vi "T7 Process Stream Data KAG.vi"(7 "Backlog":bool, 8 "error in":errorcluster, 9 "TCP Data In":string, 10 "Stream Configuration":T3={"Scan Rate (Hz)"=1000.0, "Samples Per Packet"=512, "Resolution Index"=0, "Buffer Size (bytes)"=32768, "NumScans"=1500, "Read Timeout (ms)"=5000.0, "Scan Table"=[{"Channel"=0, "BipGain"=0, "Input Config"="Single-Ended"}, {"Channel"=1, "BipGain"=0, "Input Config"="Single-Ended"}, {"Channel"=2, "BipGain"=0, "Input Config"="Single-Ended"}, {"Channel"=3, "BipGain"=0, "Input Config"="Single-Ended"}]} {"Samples Per Packet" max=512 step=1; "Buffer Size (bytes)" max=32768 step=1; "Resolution Index" max=8 step=1; "Scan Rate (Hz)" min=0.0 max=100000.0; "Scan Table"."BipGain" items=["x1", "x10", "x100", "x1000"]; "Scan Table"."Channel" step=1}, 11 "IP Configuration":T1={"Connection ID In"=refnum, "Connection ID Out"=refnum, "Device IP"="192.168.126.147", "Port"=502}) -> (0 "error out":errorcluster, 1 "Backlog Bytes":u16, 3 "Data":u16[][](array[numeric]), 5 "Packet Counter Out":i32)   [LabVIEW 2015]
doc: "Check Packet integrity and parse"
uses:
  T7 Stream Config KAG.ctl
  T7 Secondary Configs KAG.ctl
  T7 IP Config KAG.ctl
  T7 Stream Globals KAG.vi
panel:
  in  "Secondary Stream Configurations":T2={"Settling Delay (*5 us)"=0.0, "Clock Source"=0, "Auto Target"=1} {"Auto Target" max=255 step=1; "Clock Source" max=2 step=2; "Settling Delay (*5 us)" min=0.0 max=5000.0 step=1.0}
  in  "Tab Control":T4(tab)=enum."Data Array"
  out "Read Array":u8[](array[numeric]) format="%.0x"
  out "# of bytes received":i32
  out "# Bytes to Read":i32
  out "Sample Interval":dbl
  in  "Samples per Channel":i32
  out "Backlog Scans":dbl
  out "# packets":i32
  out "scans/packet":i32[](array[numeric])
  out "unsigned byte array":u8[](array[numeric])
  out "ErrorBoolean":bool
  out "Bytes / Pkt":u32
  out "Error Array":i32[][](array[numeric])
  # "29 October 2015 --\n\nI changed the VI execution from \"preallocated clone reentrant execution\" to \"Non-reentrant execution\"  while I am debugging. May want to change that back before deployment."
  # "Transaction ID"
  # "Protocol ID"
  # "Length"
  # "1 (Unit ID)"
  # "76 (Function)"
  # "Number of Samples in Current Read"
  # "Backlog"
  # "Status Code"
  # "Additional Status Info"
  # "Stream Data"
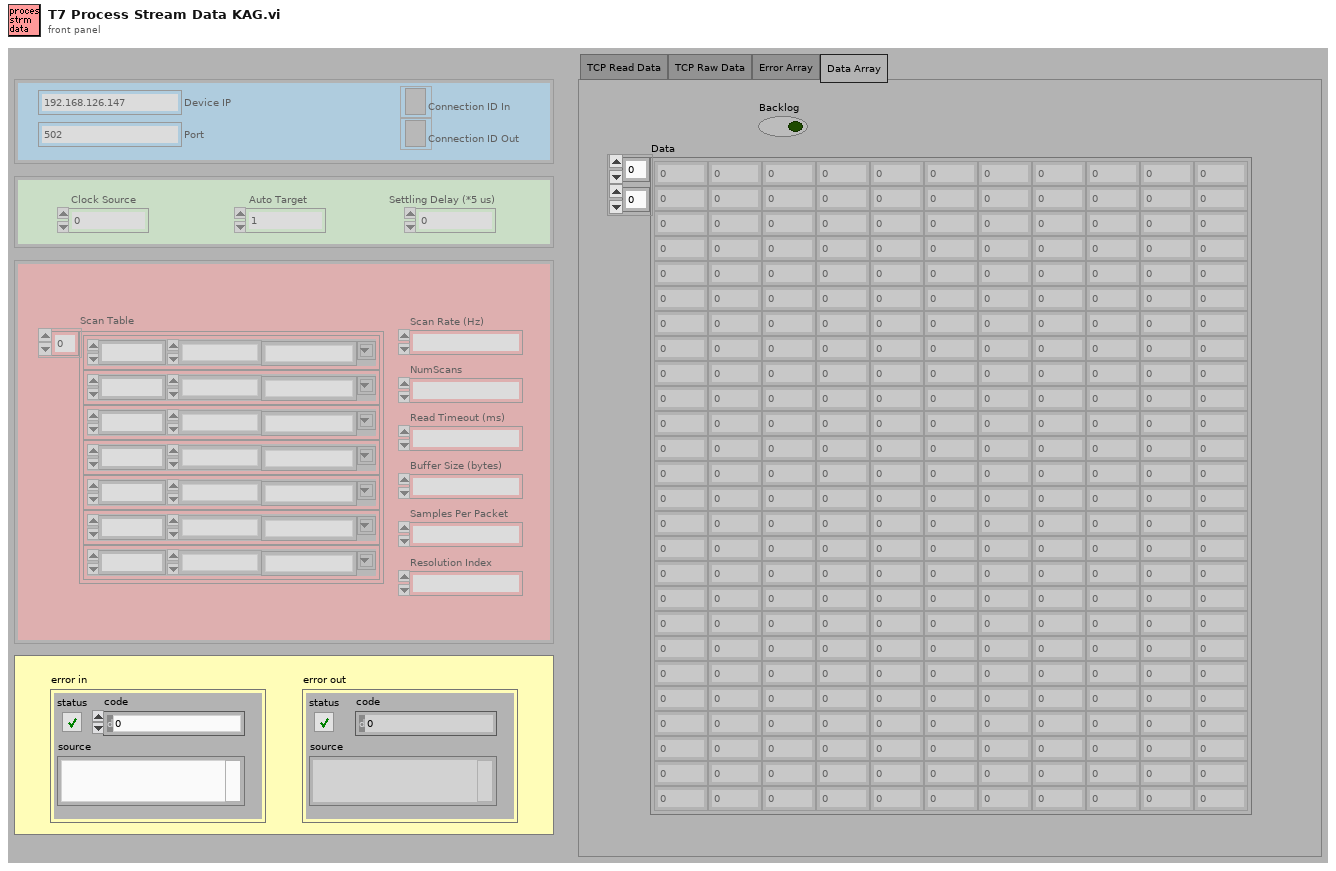
[diagram p1: front panel]
types:
  T1 = typedef "T7 IP Config KAG.ctl" = cluster{"Connection ID In":refnum<k5>, "Connection ID Out":refnum<k5>, "Device IP":string, "Port":i32}
  T2 = typedef "T7 Secondary Configs KAG.ctl" = cluster{"Settling Delay (*5 us)":dbl, "Clock Source":u32, "Auto Target":u32}
  T3 = typedef "T7 Stream Config KAG.ctl" = cluster{"Scan Rate (Hz)":dbl, "Samples Per Packet":u32, "Resolution Index":u32, "Buffer Size (bytes)":u32, "NumScans":u32, "Read Timeout (ms)":dbl, "Scan Table":cluster{"Channel":u32, "BipGain":u32, "Input Config":string}[]}
  T4 = enum32{"TCP Read Data", "TCP Raw Data", "Error Array", "Data Array"}
  T5 = cluster{"Channel":u32, "BipGain":u32, "Input Config":string}[]
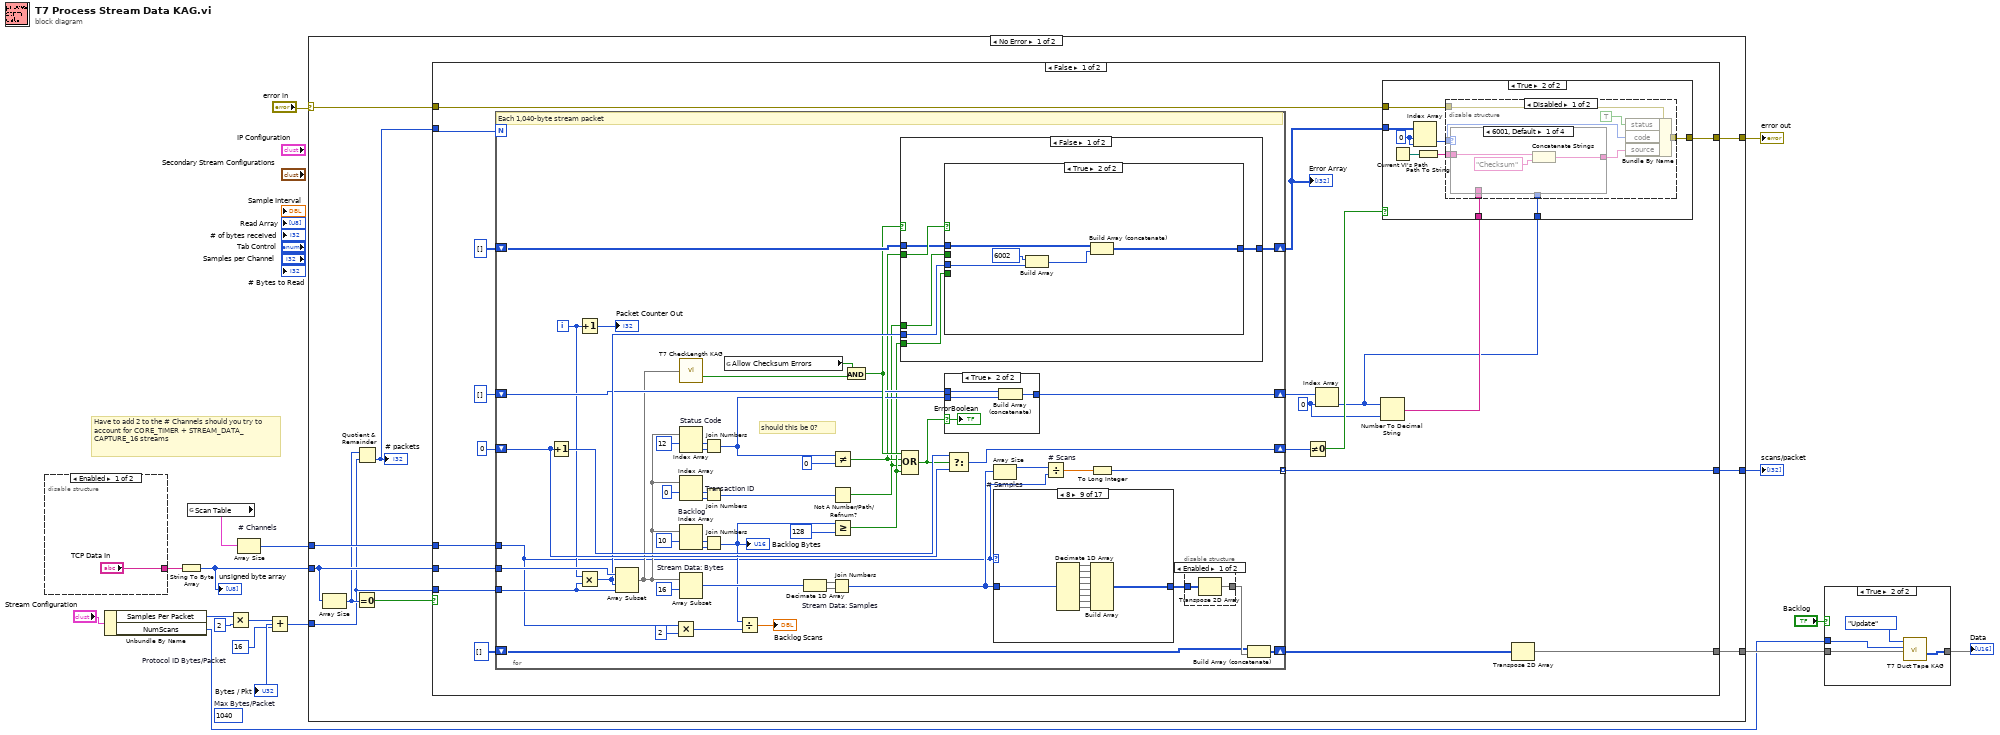
[diagram p0: block diagram]
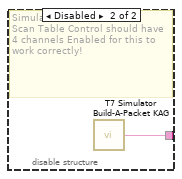
[diagram p3: hidden frame]
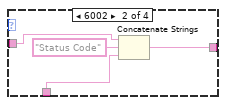
[diagram p5: hidden frame]
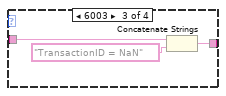
[diagram p6: hidden frame]
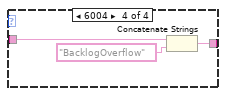
[diagram p7: hidden frame]
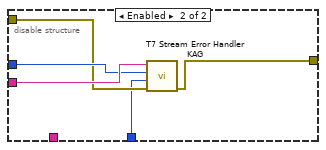
[diagram p8: hidden frame]
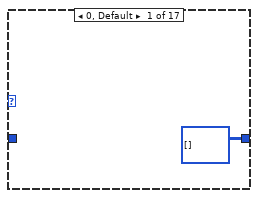
[diagram p10: hidden frame]
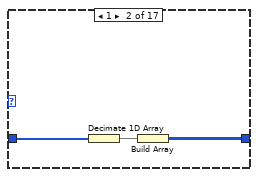
[diagram p11: hidden frame]
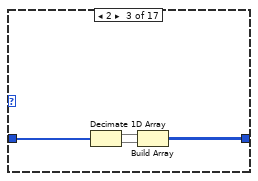
[diagram p12: hidden frame]
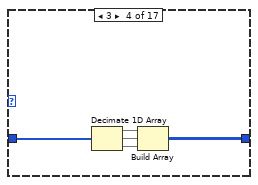
[diagram p13: hidden frame]
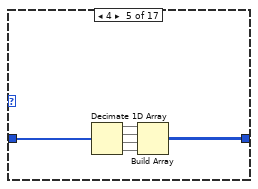
[diagram p14: hidden frame]
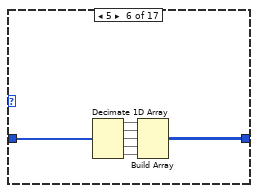
[diagram p15: hidden frame]
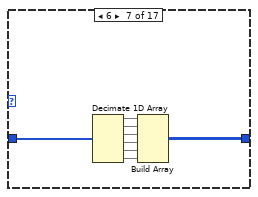
[diagram p16: hidden frame]
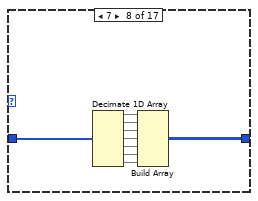
[diagram p17: hidden frame]
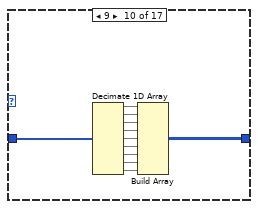
[diagram p18: hidden frame]
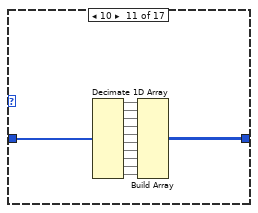
[diagram p19: hidden frame]
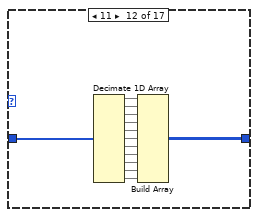
[diagram p20: hidden frame]
diagram:
  w5 = 16  # Protocol ID Bytes/Packet
  (unwired) 1040  # Max Bytes/Packet
  # "Have to add 2 to the # Channels should you try to account for CORE_TIMER + STREAM_DATA_CAPTURE_16 streams"
  n1 = disable-structure shown="Enabled" {
    disable-tunnel: ["TCP Data In" w19] -> w17
    frame Enabled {
    }
    frame Disabled {
      # "Simulate Packet\nScan Table Control should have 4 channels Enabled for this to work correctly!"
      n2 = call "T7 Simulator Build-A-Packet KAG.vi"() -> ("Simulated Data Packet"=w19:string)  [unwired: 10 in]
    }
  }
  n3 = Unbundle By Name("Stream Configuration") -> ("Samples Per Packet"=w8:u32, "NumScans"=w2:u32)
  n4 = String To Byte Array(string=w17) -> (unsigned byte array=w16:u8[])
  "unsigned byte array" <- w16
  n5 = global read "T7 Stream Globals KAG.vi" "Scan Table"() -> (w12:T5)
  n6 = Multiply(x=w8, y=2) -> (x*y=w6:u32)
  n7 = Array Size "# Channels"(array=w12) -> (size(s)=w11:i32)
  n8 = Add(x=w6, y=w5) -> (x+y=w7:u32)
  "Bytes / Pkt" <- w7
  n9 = case shown="No Error" "error in" {
    selector: "error in" -> [w29 w358]
    tunnel: [w28 w358] -> w13
    tunnel: w16 -> [w27 _]
    tunnel: w11 -> [w26 _]
    tunnel: [w25 u16[][] []] -> w4
    tunnel: w7 -> [w23 _]
    tunnel: [w21 i32[] []] -> w15
    frame No Error {
      n10 = Array Size(array=w27) -> (size(s)=w24:i32)
      n11 = Equal To 0?(x=w24) -> (x = 0?=w22:bool)
      n12 = Quotient & Remainder(x=w24, y=w23) -> (floor(x/y)=w20:u32)  [unwired: 1 out]
      "# packets" <- w20
      n13 = case shown="False" w22 {
        tunnel: w27 -> [w49 _]
        tunnel: w20 -> [w39 _]
        tunnel: w23 -> [w48 _]
        tunnel: w29 -> [w46 w352]
        tunnel: [w43 w351] -> w28
        tunnel: w26 -> [w40 _]
        tunnel: [w30 u16[][] []] -> w25
        tunnel: [w35 i32[] []] -> w21
        frame False {
          w34 = 0 ("Index")
          n14 = for {
            N: w39 -> [_]
            tunnel: w49 -> [w134]
            tunnel: w48 -> [w94]
            shift-right: [w132] -> w45
            shift-left: 0 -> [w133]
            shift-right: [w130] -> w41
            shift-left: i32[][] [] -> [w131]
            tunnel: w40 -> [w90]
            shift-right: [w119] -> w37
            shift-left: u16[] [] -> [w120]
            tunnel: [w100] -> w35 mode=indexing
            shift-right: [w86] -> w31
            shift-left: u16[][] [] -> [w85]
            i -> [w95]
            # "should this be 0?"
            # "Each 1,040-byte stream packet"
            n15 = Increment(x=w133) -> (x+1=w129:i32)
            n16 = Increment(x=w95) -> (x+1=→"Packet Counter Out":i32)
            n17 = Multiply(x=w95, y=w94) -> (x*y=w124:u32)
            n18 = Array Subset(array=w134, index=w124, length=w94) -> (w116:u8[])
            n19 = Multiply(x=w90, y=2) -> (x*y=w91:i32)
            n20 = call "T7 CheckLength KAG.vi"("Array"=w116) -> ("CheckLength Error"=w117:bool)  [unwired: 1 out]
            n21 = Index Array "Status Code"(array=w116, index #1=12 ("Index")) -> (element #1=w115:u8, element #2=w114:u8)  [unwired: 1 in]
            n22 = Index Array "Transaction ID"(array=w116, index #1=0 ("Index")) -> (element #1=w111:u8, element #2=w112:u8)  [unwired: 1 in]
            n23 = Index Array "Backlog"(array=w116, index #1=10 ("Index")) -> (element #1=w108:u8, element #2=w109:u8)  [unwired: 1 in]
            n24 = Array Subset "Stream Data: Bytes"(array=w116, index=16 ("Array Index")) -> (w107:u8[])  [unwired: 1 in]
            n25 = Join Numbers(hi=w115, lo=w114) -> ((hi.lo)=w113:u16)
            n26 = Join Numbers(hi=w111, lo=w112) -> ((hi.lo)=w110:u16)
            n27 = Join Numbers(hi=w108, lo=w109) -> ((hi.lo)=w92:u16)
            "Backlog Bytes" <- w92
            n28 = global read "T7 Stream Globals KAG.vi" "Allow Checksum Errors"() -> (w93:bool)
            n29 = Divide(x=w92, y=w91) -> (x/y=→"Backlog Scans":dbl)
            n30 = Decimate 1D Array(w107) -> (w106:u8[], w105:u8[])
            n31 = Join Numbers "Stream Data: Samples"(hi=w106, lo=w105) -> ((hi.lo)=w104:u16[])
            n32 = Not Equal?(x=w113, y=u16 0) -> (x != y?=w97:bool)
            n33 = Not A Number/Path/Refnum?(number/path/refnum=w110) -> (NaN/Path/Refnum?=w96:bool)
            n34 = Greater Or Equal?(x=w92, y=u8 128) -> (x >= y?=w98:bool)
            n35 = And(x=w93, y=w117) -> (x .and. y?=w121:bool)
            n36 = case shown="False" w121 {
              tunnel: w97 -> [w317 _]
              tunnel: w96 -> [w316 _]
              tunnel: w124 -> [w315 w346]
              tunnel: w131 -> [w313 w345]
              tunnel: [w314 w343] -> w130
              tunnel: w98 -> [w312 _]
              frame False {
                n37 = case shown="True" w317 {
                  tunnel: w316 -> [w322 _]
                  tunnel: w315 -> [w321 w340]
                  tunnel: [w319 w339] -> w314
                  tunnel: w313 -> [w320 w338]
                  tunnel: w312 -> [w318 _]
                  frame False {
                    n38 = case shown="True" w322 {
                      tunnel: w321 -> [w325 w335]
                      tunnel: w320 -> [w326 w334]
                      tunnel: [w324 w333] -> w319
                      tunnel: w318 -> [w323 _]
                      frame False {
                        n39 = case shown="True" w323 {
                          tunnel: w326 -> [w327 w330]
                          tunnel: [w327 w328] -> w324
                          tunnel: w325 -> [_ w329]
                          frame False {
                          }
                          frame True {
                            n40 = Build Array(6004, w329) -> (w331:u32[])
                            n41 = Build Array (concatenate)(w330, w331) -> (w328:u32[][])
                          }
                        }
                      }
                      frame True {
                        n42 = Build Array(6003, w335) -> (w336:u32[])
                        n43 = Build Array (concatenate)(w334, w336) -> (w333:u32[][])
                      }
                    }
                  }
                  frame True {
                    n44 = Build Array(6002, w340) -> (w341:u32[])
                    n45 = Build Array (concatenate)(w338, w341) -> (w339:u32[][])
                  }
                }
              }
              frame True {
                n46 = Build Array(6001, w346) -> (w344:u32[])
                n47 = Build Array (concatenate)(w345, w344) -> (w343:u32[][])
              }
            }
            n48 = Compound Arithmetic op=OR(w121, w97, w96, w98) -> (w122:bool)
            n49 = case shown="True" w122 {
              selector: w122 -> [_ w311]
              tunnel: w113 -> [_ w310]
              tunnel: w120 -> [w307 w309]
              tunnel: [w307 w308] -> w119
              frame False {
              }
              frame True {
                n50 = Build Array (concatenate)(w309, w310) -> (w308:u16[])
                "ErrorBoolean" <- w311
              }
            }
            n51 = Select(t=w129, s=w122, f=w133) -> (s? t:f=w132:i32)
            n52 = Array Size "# Samples"(array=w104) -> (size(s)=w102:i32)
            n53 = case shown="8" w90 {
              tunnel: w104 -> [_ w141 w145 w150 w156 w163 w171 w180 w190 w201 w213 w226 w240 w255 w271 w288 w306]
              tunnel: [u16[][] [] w139 w142 w146 w151 w157 w164 w172 w181 w191 w202 w214 w227 w242 w258 w275 w293] -> w103
              frame 0, Default {
              }
              frame 1 {
                n54 = Decimate 1D Array(w141) -> (w140:u16[])
                n55 = Build Array(w140) -> (w139:u16[][])
              }
              frame 2 {
                n56 = Decimate 1D Array(w145) -> (w144:u16[], w143:u16[])
                n57 = Build Array(w144, w143) -> (w142:u16[][])
              }
              frame 3 {
                n58 = Decimate 1D Array(w150) -> (w149:u16[], w148:u16[], w147:u16[])
                n59 = Build Array(w149, w148, w147) -> (w146:u16[][])
              }
              frame 4 {
                n60 = Decimate 1D Array(w156) -> (w155:u16[], w154:u16[], w153:u16[], w152:u16[])
                n61 = Build Array(w155, w154, w153, w152) -> (w151:u16[][])
              }
              frame 5 {
                n62 = Decimate 1D Array(w163) -> (w162:u16[], w161:u16[], w160:u16[], w159:u16[], w158:u16[])
                n63 = Build Array(w162, w161, w160, w159, w158) -> (w157:u16[][])
              }
              frame 6 {
                n64 = Decimate 1D Array(w171) -> (w170:u16[], w169:u16[], w168:u16[], w167:u16[], w166:u16[], w165:u16[])
                n65 = Build Array(w170, w169, w168, w167, w166, w165) -> (w164:u16[][])
              }
              frame 7 {
                n66 = Decimate 1D Array(w180) -> (w179:u16[], w178:u16[], w177:u16[], w176:u16[], w175:u16[], w174:u16[], w173:u16[])
                n67 = Build Array(w179, w178, w177, w176, w175, w174, w173) -> (w172:u16[][])
              }
              frame 8 {
                n68 = Decimate 1D Array(w190) -> (w189:u16[], w188:u16[], w187:u16[], w186:u16[], w185:u16[], w184:u16[], w183:u16[], w182:u16[])
                n69 = Build Array(w189, w188, w187, w186, w185, w184, w183, w182) -> (w181:u16[][])
              }
              frame 9 {
                n70 = Decimate 1D Array(w201) -> (w200:u16[], w199:u16[], w198:u16[], w197:u16[], w196:u16[], w195:u16[], w194:u16[], w193:u16[], w192:u16[])
                n71 = Build Array(w200, w199, w198, w197, w196, w195, w194, w193, w192) -> (w191:u16[][])
              }
              frame 10 {
                n72 = Decimate 1D Array(w213) -> (w212:u16[], w211:u16[], w210:u16[], w209:u16[], w208:u16[], w207:u16[], w206:u16[], w205:u16[], w204:u16[], w203:u16[])
                n73 = Build Array(w212, w211, w210, w209, w208, w207, w206, w205, w204, w203) -> (w202:u16[][])
              }
              frame 11 {
                n74 = Decimate 1D Array(w226) -> (w225:u16[], w224:u16[], w223:u16[], w222:u16[], w221:u16[], w220:u16[], w219:u16[], w218:u16[], w217:u16[], w216:u16[], w215:u16[])
                n75 = Build Array(w225, w224, w223, w222, w221, w220, w219, w218, w217, w216, w215) -> (w214:u16[][])
              }
              frame 12 {
                n76 = Decimate 1D Array(w240) -> (w239:u16[], w238:u16[], w237:u16[], w236:u16[], w235:u16[], w234:u16[], w233:u16[], w232:u16[], w231:u16[], w230:u16[], w229:u16[], w228:u16[])
                n77 = Build Array(w239, w238, w237, w236, w235, w234, w233, w232, w231, w230, w229, w228) -> (w227:u16[][])
              }
              frame 13 {
                n78 = Decimate 1D Array(w255) -> (w254:u16[], w253:u16[], w252:u16[], w251:u16[], w250:u16[], w249:u16[], w248:u16[], w247:u16[], w246:u16[], w245:u16[], w244:u16[], w243:u16[], w241:u16[])
                n79 = Build Array(w254, w253, w252, w251, w250, w249, w248, w247, w246, w245, w244, w243, w241) -> (w242:u16[][])
              }
              frame 14 {
                # "Unless AI is expanded with MUX 80, max AIN = 14"
                n80 = Decimate 1D Array(w271) -> (w270:u16[], w269:u16[], w268:u16[], w267:u16[], w266:u16[], w265:u16[], w264:u16[], w263:u16[], w262:u16[], w261:u16[], w260:u16[], w259:u16[], w257:u16[], w256:u16[])
                n81 = Build Array(w270, w269, w268, w267, w266, w265, w264, w263, w262, w261, w260, w259, w257, w256) -> (w258:u16[][])
              }
              frame 15 {
                # "Added this to account for CORE_TIMER stream"
                n82 = Decimate 1D Array(w288) -> (w287:u16[], w286:u16[], w285:u16[], w284:u16[], w283:u16[], w282:u16[], w281:u16[], w280:u16[], w279:u16[], w278:u16[], w277:u16[], w276:u16[], w274:u16[], w273:u16[], w272:u16[])
                n83 = Build Array(w287, w286, w285, w284, w283, w282, w281, w280, w279, w278, w277, w276, w274, w273, w272) -> (w275:u16[][])
              }
              frame 16 {
                # "Added this to account for STREAM_DATA_CAPTURE_16 stream"
                n84 = Decimate 1D Array(w306) -> (w305:u16[], w304:u16[], w303:u16[], w302:u16[], w301:u16[], w300:u16[], w299:u16[], w298:u16[], w297:u16[], w296:u16[], w295:u16[], w294:u16[], w292:u16[], w291:u16[], w290:u16[], w289:u16[])
                n85 = Build Array(w305, w304, w303, w302, w301, w300, w299, w298, w297, w296, w295, w294, w292, w291, w290, w289) -> (w293:u16[][])
              }
            }
            n86 = Divide "# Scans"(x=w102, y=w90) -> (x/y=w101:dbl)
            n87 = To Long Integer(number=w101) -> (32bit integer=w100:i32)
            n88 = disable-structure shown="Enabled" {
              disable-tunnel: w103 -> [w136 w137]
              disable-tunnel: [w135 w137] -> w87
              frame Enabled {
                n89 = Transpose 2D Array(2D array=w136) -> (transposed array=w135:u16[][])
              }
              frame Disabled {
              }
            }
            n90 = Build Array (concatenate)(w85, w87) -> (w86:u16[][])
          }
          "Error Array" <- w41
          n91 = Not Equal To 0?(x=w45) -> (x != 0?=w44:bool)
          n92 = Index Array(array=w37, index=w34) -> (element=w33:u16)
          n93 = Number To Decimal String(number=w33, width (-)=w34) -> (decimal integer string=w36:string)
          n94 = case shown="True" w44 {
            tunnel: w46 -> [w50 w54]
            tunnel: [w50 w55] -> w43
            tunnel: w41 -> [_ w59]
            tunnel: w36 -> [_ w53]
            tunnel: w33 -> [_ w51]
            frame False {
            }
            frame True {
              w58 = 0 ("Index (row)")
              n95 = Current VI's Path() -> (path=w57:path)
              n96 = Index Array(array=w59, index (row)=w58, index (col)=w58) -> (element=w52:u32)
              n97 = Path To String(path=w57) -> (string=w56:string)
              n98 = disable-structure shown="Disabled" {
                disable-tunnel: w56 -> [w65 w84]
                disable-tunnel: [w63 w81] -> w55
                disable-tunnel: w54 -> [w62 w82]
                disable-tunnel: w53 -> [w61 _]
                disable-tunnel: w52 -> [w60 w83]
                disable-tunnel: w51 -> [_ w80]
                frame Disabled {
                  n99 = case shown="6001, Default" w60 {
                    tunnel: w65 -> [w68 w73 w76 w79]
                    tunnel: [w67 w71 w74 w77] -> w64
                    tunnel: w61 -> [_ w70 _ _]
                    frame 6001, Default {
                      n100 = Concatenate Strings(w68, "Checksum" ("Substring")) -> (w67:string)
                    }
                    frame 6002 {
                      n101 = Concatenate Strings(w73, "Status Code" ("Substring"), w70) -> (w71:string)
                    }
                    frame 6003 {
                      n102 = Concatenate Strings(w76, "TransactionID = NaN" ("Substring")) -> (w74:string)
                    }
                    frame 6004 {
                      n103 = Concatenate Strings(w79, "BacklogOverflow" ("Substring")) -> (w77:string)
                    }
                  }
                  n104 = Bundle By Name(cluster=w62, "status"=TRUE, "code"=w60, "source"=w64) -> (w63:errorcluster)
                }
                frame Enabled {
                  n105 = call "T7 Stream Error Handler KAG.vi"("error in"=w82, "Status Code"=w80, "Error Code"=w83, "Error Source"=w84) -> ("error out"=w81:errorcluster)  [unwired: 7 in]
                }
              }
            }
          }
          n106 = Transpose 2D Array(2D array=w31) -> (transposed array=w30:u16[][])
        }
        frame True {
          n107 = Current VI's Path() -> (path=w354:path)
          n108 = Path To String(path=w354) -> (string=w353:string)
          n109 = Bundle By Name(cluster=w352, "status"=TRUE, "code"=u32 6000 ("y"), "source"=w353) -> (w351:errorcluster)
        }
      }
    }
    frame Error {
    }
  }
  "scans/packet" <- w15
  "error out" <- w13
  n110 = case shown="True" "Backlog" {
    tunnel: w4 -> [w359 w363]
    tunnel: [w359 w362] -> w3
    tunnel: w2 -> [_ w361]
    frame False {
    }
    frame True {
      n111 = call "T7 Duct Tape KAG.vi"("incoming"=w363, "NumScans requested"=w361, "Action"=enum16{"Initialize", "Read", "Update"}."Update") -> ("requested"=w362:u16[][])  [unwired: 6 in]
    }
  }
  "Data" <- w3
